vi "CalculateAntsRect.vi"(9 "AntsRect":T2, 10 "Mouse Down Coords":T1, 11 "Mouse Move Coords":T1) -> (2 "Rect":cluster{i32, i32, i32, i32})   [LabVIEW 2021]
uses:
  <vilib>/Utility/miscctls.llb/LVPoint32TypeDef.ctl
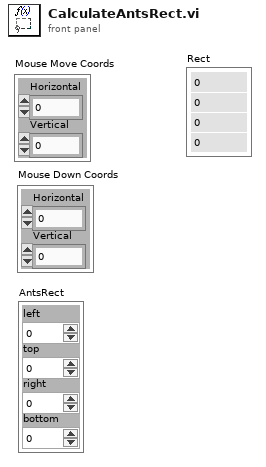
[diagram p1: front panel]
types:
  T1 = typedef "LVPoint32TypeDef.ctl" = cluster{"Horizontal":i32, "Vertical":i32}
  T2 = cluster{"left":i16, "top":i16, "right":i16, "bottom":i16}
  T3 = cluster{"Horizontal":i32, "Vertical":i32, "Horizontal":i32, "Vertical":i32}
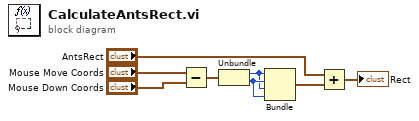
[diagram p0: block diagram]
diagram:
  n1 = Subtract(x="Mouse Move Coords", y="Mouse Down Coords") -> (x-y=w1:T1)
  n2 = Unbundle(w1) -> ("Horizontal"=w2:i32, "Vertical"=w3:i32)
  n3 = Bundle("Horizontal"=w2, "Vertical"=w3, "Horizontal"=w2, "Vertical"=w3) -> (w4:T3)  [unwired: 1 out]
  n4 = Add(x="AntsRect", y=w4) -> (x+y=→"Rect":cluster{i32, i32, i32, i32})
